vi "Create.vi"(8 "error in (no error)":errorcluster, 9 "ID":i32, 10 "Name":string, 11 "Motor in":refnum<class "Motor-Sieve.lvclass">) -> (0 "error out":errorcluster, 3 "Motor out":refnum<class "Motor-Sieve.lvclass">)   [LabVIEW 2013, in "PowderDeposition.lvlib" / "Motor-Sieve.lvclass"]
uses:
  Motor-Sieve.lvclass
  Units.ctl
  Action-settings.ctl
  Motor-Analog.lvclass/Motor-Analog.ctl
  Write Maximum speed.vi
  Write Maximum value.vi
  Write Minimum speed.vi
  Write Minimum value.vi
  Write Motor DAQ channel.vi
  Write Maximum voltage.vi
  Write Speed factor.vi
  Motor.lvclass
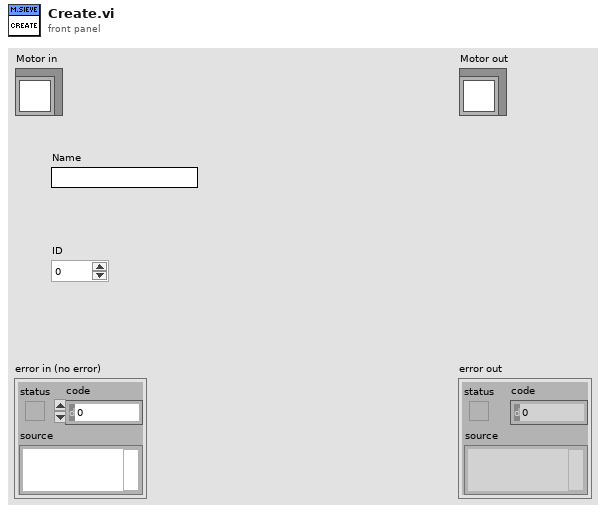
[diagram p1: front panel]
types:
  T1 = typedef "PowderDeposition.lvlib/Motor.lvclass/Action-settings.ctl" = cluster{"Speed":dbl, "Acceleration":dbl, "Direction":enum16{"Clockwise", "Counter-clockwise"}}
  T2 = typedef "PowderDeposition.lvlib/Motor.lvclass/Units.ctl" = enum16{"-", "mm", "µm", "tr", "V"}
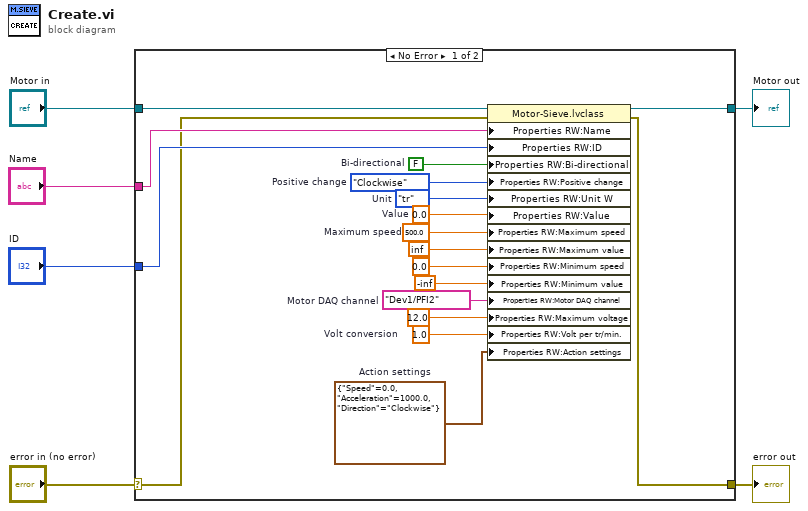
[diagram p0: block diagram]
diagram:
  n1 = case shown="No Error" "error in (no error)" {
    selector: "error in (no error)" -> [w7 w26]
    tunnel: [w8 w26] -> w5
    tunnel: [w9 w25] -> w3
    tunnel: "Motor in" -> [w24 w25]
    tunnel: "Name" -> [w23 _]
    tunnel: "ID" -> [w22 _]
    frame No Error {
      w10 = T1 {"Speed"=0.0, "Acceleration"=1000.0, "Direction"=enum."Clockwise"}  # Action settings
      w11 = tag "Dev1/PFI2"  # Motor DAQ channel
      w12 = 1.0  # Volt conversion
      w17 = 500.0  # Maximum speed
      w18 = 0.0  # Value
      w19 = Units."tr"  # Unit
      w20 = enum16{"Clockwise", "Counter-clockwise"}."Clockwise"  # Positive change
      w21 = FALSE  # Bi-directional
      n2 = property class="Motor-Sieve.lvclass"(reference=w24, error in=w7, "Properties RW:Name"=w23, "Properties RW:ID"=w22, "Properties RW:Bi-directional"=w21, "Properties RW:Positive change"=w20, "Properties RW:Unit W"=w19, "Properties RW:Value"=w18, "Properties RW:Maximum speed"=w17, "Properties RW:Maximum value"=inf, "Properties RW:Minimum speed"=0.0 ("Minimum voltage"), "Properties RW:Minimum value"=-inf, "Properties RW:Motor DAQ channel"=w11, "Properties RW:Maximum voltage"=12.0 ("Volt per tr/min."), "Properties RW:Volt per tr/min."=w12, "Properties RW:Action settings"=w10) -> (reference out=w9:refnum<class "Motor-Sieve.lvclass">, error out=w8:errorcluster)
    }
    frame Error {
    }
  }
  "error out" <- w5
  "Motor out" <- w3
